vi "Find and Shift SMPS sizes according to selected Peak Position.vi"(6 "Sizes":dbl[](array[numeric]), 9 "SMPS Sizes":dbl[](array[numeric]), 10 "Concentration":dbl[][](array[numeric]), 11 "method":i32) -> (1 "Peak Position in the old data":dbl[](array[numeric]), 2 "SMPS sizes":dbl[](array[numeric]), 3 "Shifted Concentration":dbl[][](array[numeric]))   [LabVIEW 2013]
doc: "Finds peaks of main size distribution. \nCompares to selected sizes\nshifts the whole distributions, such that the main peak will exactly on top of the selected size peak\nReturns shifted peak. SMPS sizes are unchanged."
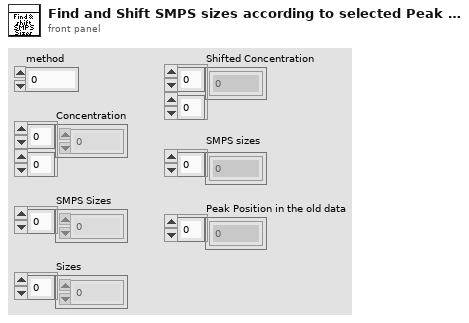
[diagram p1: front panel]
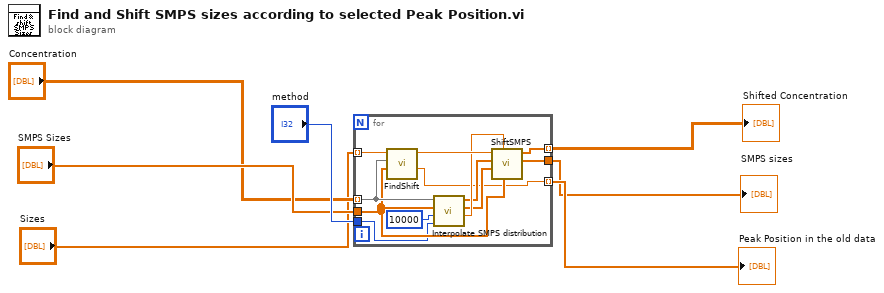
[diagram p0: block diagram]
diagram:
  n1 = for {
    tunnel: "Concentration" -> [w18] mode=indexing
    tunnel: "SMPS Sizes" -> [w12]
    tunnel: "Sizes" -> [w14] mode=indexing
    tunnel: [w11] -> w7 mode=indexing
    tunnel: [w10] -> w1
    tunnel: "method" -> [w9]
    tunnel: [w8] -> w6 mode=indexing
    n2 = call "FindShift.vi"("SMPS Sizes"=w12, "Concentration"=w18, "Sizes"=w14) -> ("Peak Center"=w8:dbl, "Shift in Log scale"=w17:dbl)  [unwired: 6 in, 1 out]
    n3 = call "Interpolate SMPS distribution.vi"("method"=w9, "samples"=10000, "SMPS Sizes"=w12, "Concentration"=w18) -> ("DeltaX"=w16:dbl, "xi used"=w13:dbl[], "yi"=w15:dbl[])  [unwired: 5 in]
    n4 = call "ShiftSMPS.vi"("SMPS Sizes"=w12, "DeltaX"=w16, "xi used in"=w13, "yi in"=w15, "Shift in Log scale"=w17) -> ("xi used out"=w10:dbl[], "yi out"=w11:dbl[])  [unwired: 5 in]
  }
  "Shifted Concentration" <- w7
  "Peak Position in the old data" <- w6
  "SMPS sizes" <- w1
